vi "SwitchOption.vi"(6 "SubPanelRef":refnum<vi>, 7 "Panel Controller":refnum<class "MemberPanel.lvclass">, 8 "error in (no error)":errorcluster, 9 "Base Path":path, 10 "ThreadName(\"\")":string, 11 "Admin_Actor in":refnum<class "Admin_Actor.lvclass">) -> (0 "error out":errorcluster, 3 "Admin_Actor out":refnum<class "Admin_Actor.lvclass">)   [LabVIEW 2015, in "Admin_Actor.lvlib" / "Admin_Actor.lvclass"]
uses:
  Admin_Actor.lvclass
  Member_Actor/MemberPanel/MemberPanel.lvclass
  Admin_Actor.lvclass/Admin_Actor.ctl
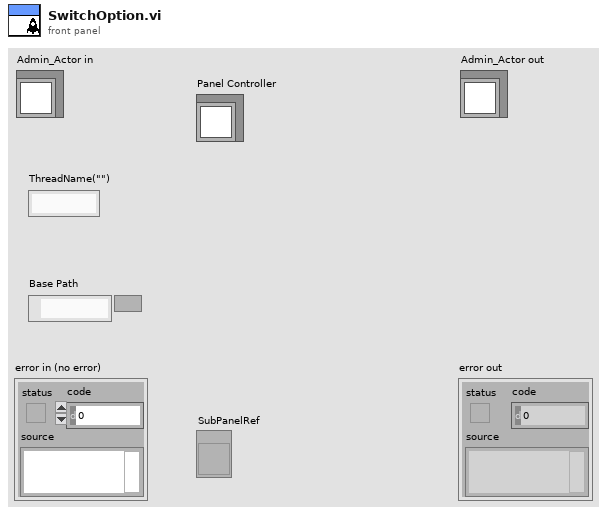
[diagram p1: front panel]
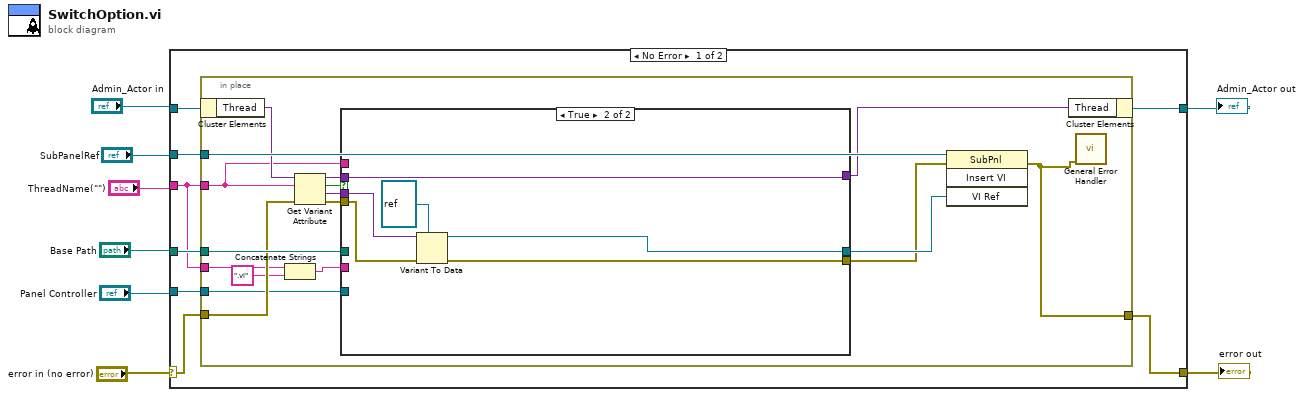
[diagram p0: block diagram]
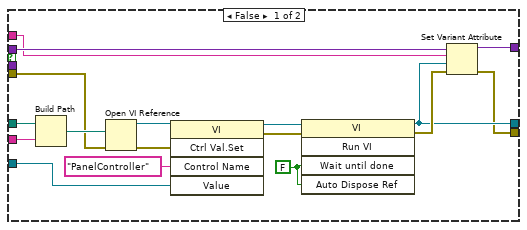
[diagram p2: hidden frame]
diagram:
  n1 = case shown="No Error" "error in (no error)" {
    selector: "error in (no error)" -> [w11 w58]
    tunnel: [w14 w58] -> w4
    tunnel: [w10 w57] -> w1
    tunnel: "Admin_Actor in" -> [w13 w57]
    tunnel: "Base Path" -> [w16 _]
    tunnel: "ThreadName(\"\")" -> [w12 _]
    tunnel: "SubPanelRef" -> [w15 _]
    tunnel: "Panel Controller" -> [w9 _]
    frame No Error {
      n2 = in-place {
        in-place-border: w16 -> [w33]
        in-place-border: w12 -> [w21]
        in-place-border: w15 -> [w32]
        in-place-border: [w18] -> w14
        in-place-border: w12 -> [w17]
        in-place-border: w11 -> [w28]
        in-place-border: w9 -> [w22]
        n3 = in-place-cluster #1(w13) -> ("Thread"=w29:variant)
        n4 = Concatenate Strings(w21, ".vi" ("string")) -> (w19:string)
        n5 = Get Variant Attribute(Variant=w29, name=w17, error in=w28) -> (duplicate Variant=w25:variant, found=w27:bool, value=w24:variant, error out=w26:errorcluster)  [unwired: 1 in]
        n6 = case shown="True" w27 {
          tunnel: w33 -> [w50 _]
          tunnel: w19 -> [w43 _]
          tunnel: [w44 w53] -> w31
          tunnel: [w42 w52] -> w30
          tunnel: w26 -> [w47 w55]
          tunnel: w25 -> [w46 w51]
          tunnel: [w41 w51] -> w23
          tunnel: w24 -> [_ w56]
          tunnel: w22 -> [w35 _]
          tunnel: w17 -> [w34 _]
          frame False {
            w48 = FALSE ("Wait Until Done")
            n7 = Build Path(base path=w50, name or relative path=w43) -> (appended path=w49:path)
            n8 = Open VI Reference(vi path=w49, error in (no error)=w47) -> (vi reference=w40:refnum<vi>, error out=w39:errorcluster)  [unwired: 4 in]
            n9 = invoke class="VI" method="Ctrl Val.Set"(reference=w40, error in=w39, "Control Name"="PanelController", "Value"=w35) -> (reference out=w37:refnum<vi>, error out=w38:errorcluster)  [unwired: 1 in, 3 out]
            n10 = invoke class="VI" method="Run VI"(reference=w37, error in=w38, "Wait until done"=w48, "Auto Dispose Ref"=w48) -> (reference out=w44:refnum<vi>, error out=w45:errorcluster)  [unwired: 1 in, 3 out]
            n11 = Set Variant Attribute(Variant=w46, name=w34, value=w44, error in=w45) -> (Variant out=w41:variant, error out=w42:errorcluster)  [unwired: 1 out]
          }
          frame True {
            n12 = Variant To Data(error in=w55, type=refnum<vi> refnum ("vi reference"), Variant=w56) -> (data=w53:refnum<vi>, error out=w52:errorcluster)
          }
        }
        n13 = invoke class="SubPnl" method="Insert VI"(reference=w32, error in=w30, "VI Ref"=w31) -> (error out=w18:errorcluster)  [unwired: 1 in, 3 out]
        n14 = in-place-cluster #1("Thread"=w23) -> (w10:refnum<class "Admin_Actor.lvclass">)
        n15 = call <vilib>:"General Error Handler.vi"("error in (no error)"=w18) -> ()  [unwired: 10 in, 5 out]
      }
    }
    frame Error {
    }
  }
  "error out" <- w4
  "Admin_Actor out" <- w1
